vi "Start Command.vi"(8 "error in (no error)":errorcluster, 11 "Command in":refnum<class "Command Actor.lvclass">) -> (0 "error out":errorcluster, 3 "Command out":refnum<class "Command Actor.lvclass">)   [LabVIEW 2014, in "Robot Actor Framework.lvlib" / "Command Actor.lvlib" / "Command Actor.lvclass"]
uses:
  Command Actor.lvclass
  Command States.ctl
  <vilib>/ActorFramework/Message Enqueuer/Message Priority.ctl
  Command Actor.lvclass/Command Actor.ctl
  <vilib>/ActorFramework/Actor/Actor.lvclass/Actor.ctl
  Command Processor Actor/Command Processor Actor Messages/Command Started Msg/Command Started Msg.lvclass/Command Started Msg.ctl
  <vilib>/ActorFramework/Message Enqueuer/Message Enqueuer.lvclass/Message Enqueuer.ctl
  <vilib>/ActorFramework/Message Enqueuer/Enqueue.vi
  <vilib>/ActorFramework/Message Priority Queue/Priority Enqueue.vi
  Command Processor Actor/Command Processor Actor Messages/Command Started Msg/Command Started Msg.lvclass
  <vilib>/ActorFramework/Actor/Actor.lvclass
  <vilib>/ActorFramework/Message Enqueuer/Message Enqueuer.lvclass
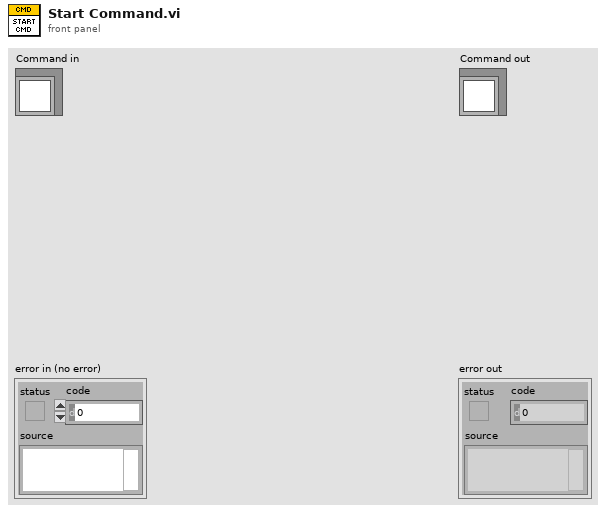
[diagram p1: front panel]
types:
  T1 = typedef "Actor Framework.lvlib/Message Enqueuer.lvclass/Message Priority.ctl" = enum16{"Low", "Normal", "High"}
  T2 = enum16{"Critical", "Error", "Warning", "Informational", "Debug"}
  T3 = typedef "Robot Actor Framework.lvlib/Command Actor.lvlib/Command Actor.lvclass/Command States.ctl" = enum16{"Unknown", "Started", "Stopped", "Finished"}
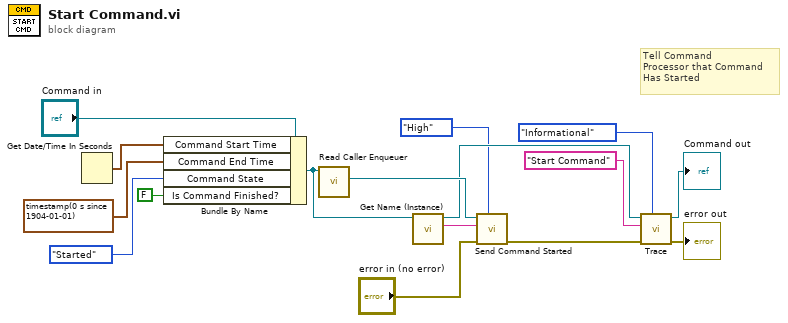
[diagram p0: block diagram]
diagram:
  # "Tell Command\nProcessor that Command\nHas Started"
  n1 = Get Date/Time In Seconds() -> (seconds since 1Jan1904=w11:timestamp)
  n2 = Bundle By Name(cluster="Command in", "Command Start Time"=w11, "Command End Time"=timestamp(0 s since 1904-01-01), "Command State"=Command_States."Started", "Is Command Finished?"=FALSE) -> (w4:refnum<class "Command Actor.lvclass">)
  n3 = call <vilib>:"Read Caller Enqueuer.vi"("Actor"=w4) -> ("Caller Enqueuer"=w12:refnum<class "Message Enqueuer.lvclass">)  [unwired: 10 in]
  n4 = call-dynamic "Get Name (Instance).vi"("Command Actor in"=w4) -> ("Name (Instance)"=w3:string, "Command Actor out"=w2:refnum<class "Command Actor.lvclass">)  [unwired: 8 in, 1 out]
  n5 = call "Send Command Started.vi"("Message Priority (Normal)"=Message_Priority."High", "error in (no error)"="error in (no error)", "Command Name (Instance)"=w3, "Message Enqueuer"=w12) -> ("error out"=w5:errorcluster)  [unwired: 6 in, 1 out]
  n6 = call-dynamic "Trace.vi"("Trace Level"=T2."Informational", "error in (no error)"=w5, "Command Action"="Start Command", "Command Actor in"=w2) -> ("error out"=→"error out":errorcluster, "Command Actor out"=→"Command out":refnum<class "Command Actor.lvclass">)  [unwired: 6 in]
